vi "Guess library path.vi"() -> (2 "paths":path[](array[path]))   [LabVIEW 2020, in "lvzstd.lvlib"]
uses:
  lvzstd.lvlib
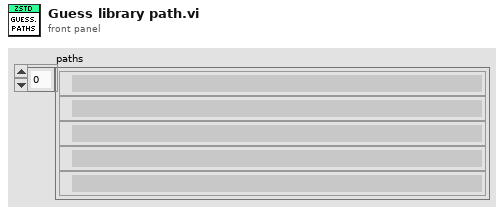
[diagram p1: front panel]
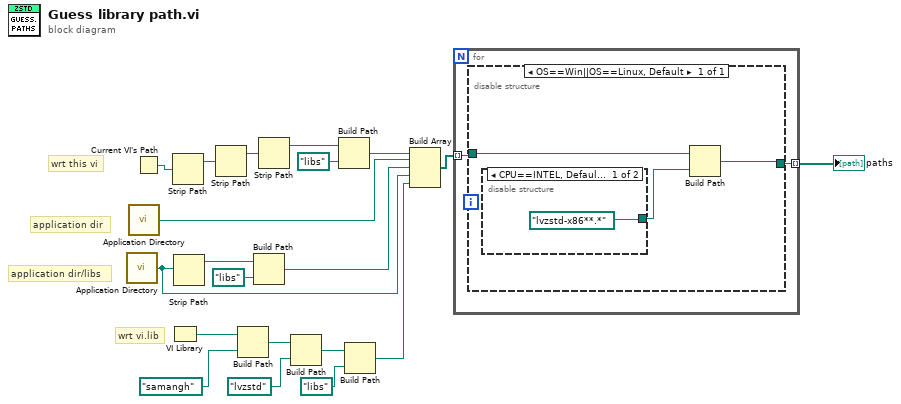
[diagram p0: block diagram]
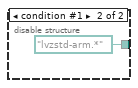
[diagram p2: hidden frame]
diagram:
  # "application dir/libs"
  # "wrt vi.lib"
  # "application dir"
  # "wrt this vi"
  n1 = call <vilib>:"Application Directory.vi"() -> ("Application Directory"=w3:path)
  n2 = call <vilib>:"Application Directory.vi"() -> ("Application Directory"=w1:path)
  n3 = Current VI's Path() -> (path=w11:path)
  n4 = VI Library() -> (path=w10:path)
  n5 = Strip Path(path=w11) -> (stripped path=w20:path)  [unwired: 1 out]
  n6 = Strip Path(path=w3) -> (stripped path=w15:path)  [unwired: 1 out]
  n7 = Strip Path(path=w20) -> (stripped path=w19:path)  [unwired: 1 out]
  n8 = Build Path(base path=w10, name or relative path=path "samangh") -> (appended path=w8:path)
  n9 = Build Path(base path=w15, name or relative path=path "libs") -> (appended path=w2:path)
  n10 = Strip Path(path=w19) -> (stripped path=w18:path)  [unwired: 1 out]
  n11 = Build Path(base path=w8, name or relative path=path "lvzstd") -> (appended path=w5:path)
  n12 = Build Path(base path=w18, name or relative path=path "libs") -> (appended path=w14:path)
  n13 = Build Path(base path=w5, name or relative path=path "libs") -> (appended path=w4:path)
  n14 = Build Array(w14, w1, w2, w3, w4) -> (w13:path[])
  n15 = for {
    tunnel: w13 -> [w22] mode=indexing
    tunnel: [w21] -> w12 mode=indexing
    n16 = disable-structure shown="OS==Win||OS==Linux, Default" {
      disable-tunnel: w22 -> [w25]
      disable-tunnel: [w24] -> w21
      frame condition #0 (active) {
        n17 = disable-structure shown="CPU==INTEL, Default" {
          disable-tunnel: [path "lvzstd-x86**.*" ("name or relative path") path "lvzstd-arm.*" ("name or relative path")] -> w23
          frame condition #0 (active) {
          }
          frame condition #1 {
          }
        }
        n18 = Build Path(base path=w25, name or relative path=w23) -> (appended path=w24:path)
      }
    }
  }
  "paths" <- w12
